vi "PumpValve4.vi"() -> ()   [LabVIEW 2015]
uses:
  PumpValve.ctl
  <vilib>/DAQmx/write.llb/DAQmx Write (Digital 1D Bool NChan 1Samp 1Line).vi
  <vilib>/DAQmx/miscellaneous.llb/DAQmx Fill In Error Info.vi
panel:
  in  "Duty cycle % (0-100)":dbl=50.0
  in  "stop":bool
  in  "Steps in a cycle":i32=256
  in  "Cycle time (s)":i32=5
  in  "On/Off (Pump)":bool
  in  "Open/Close (Blue)":bool
  in  "Open/Close (Green)":bool
  in  "Manual Mode":bool
  out "Invalid fill%":bool
  out "Tank":u32(slide) scale=0.0..100.0
  in  "Drain %":u32
  in  "Fill %":u32
  in  "Drain":bool
  in  "Stop Program":bool
  in  "Fill":bool
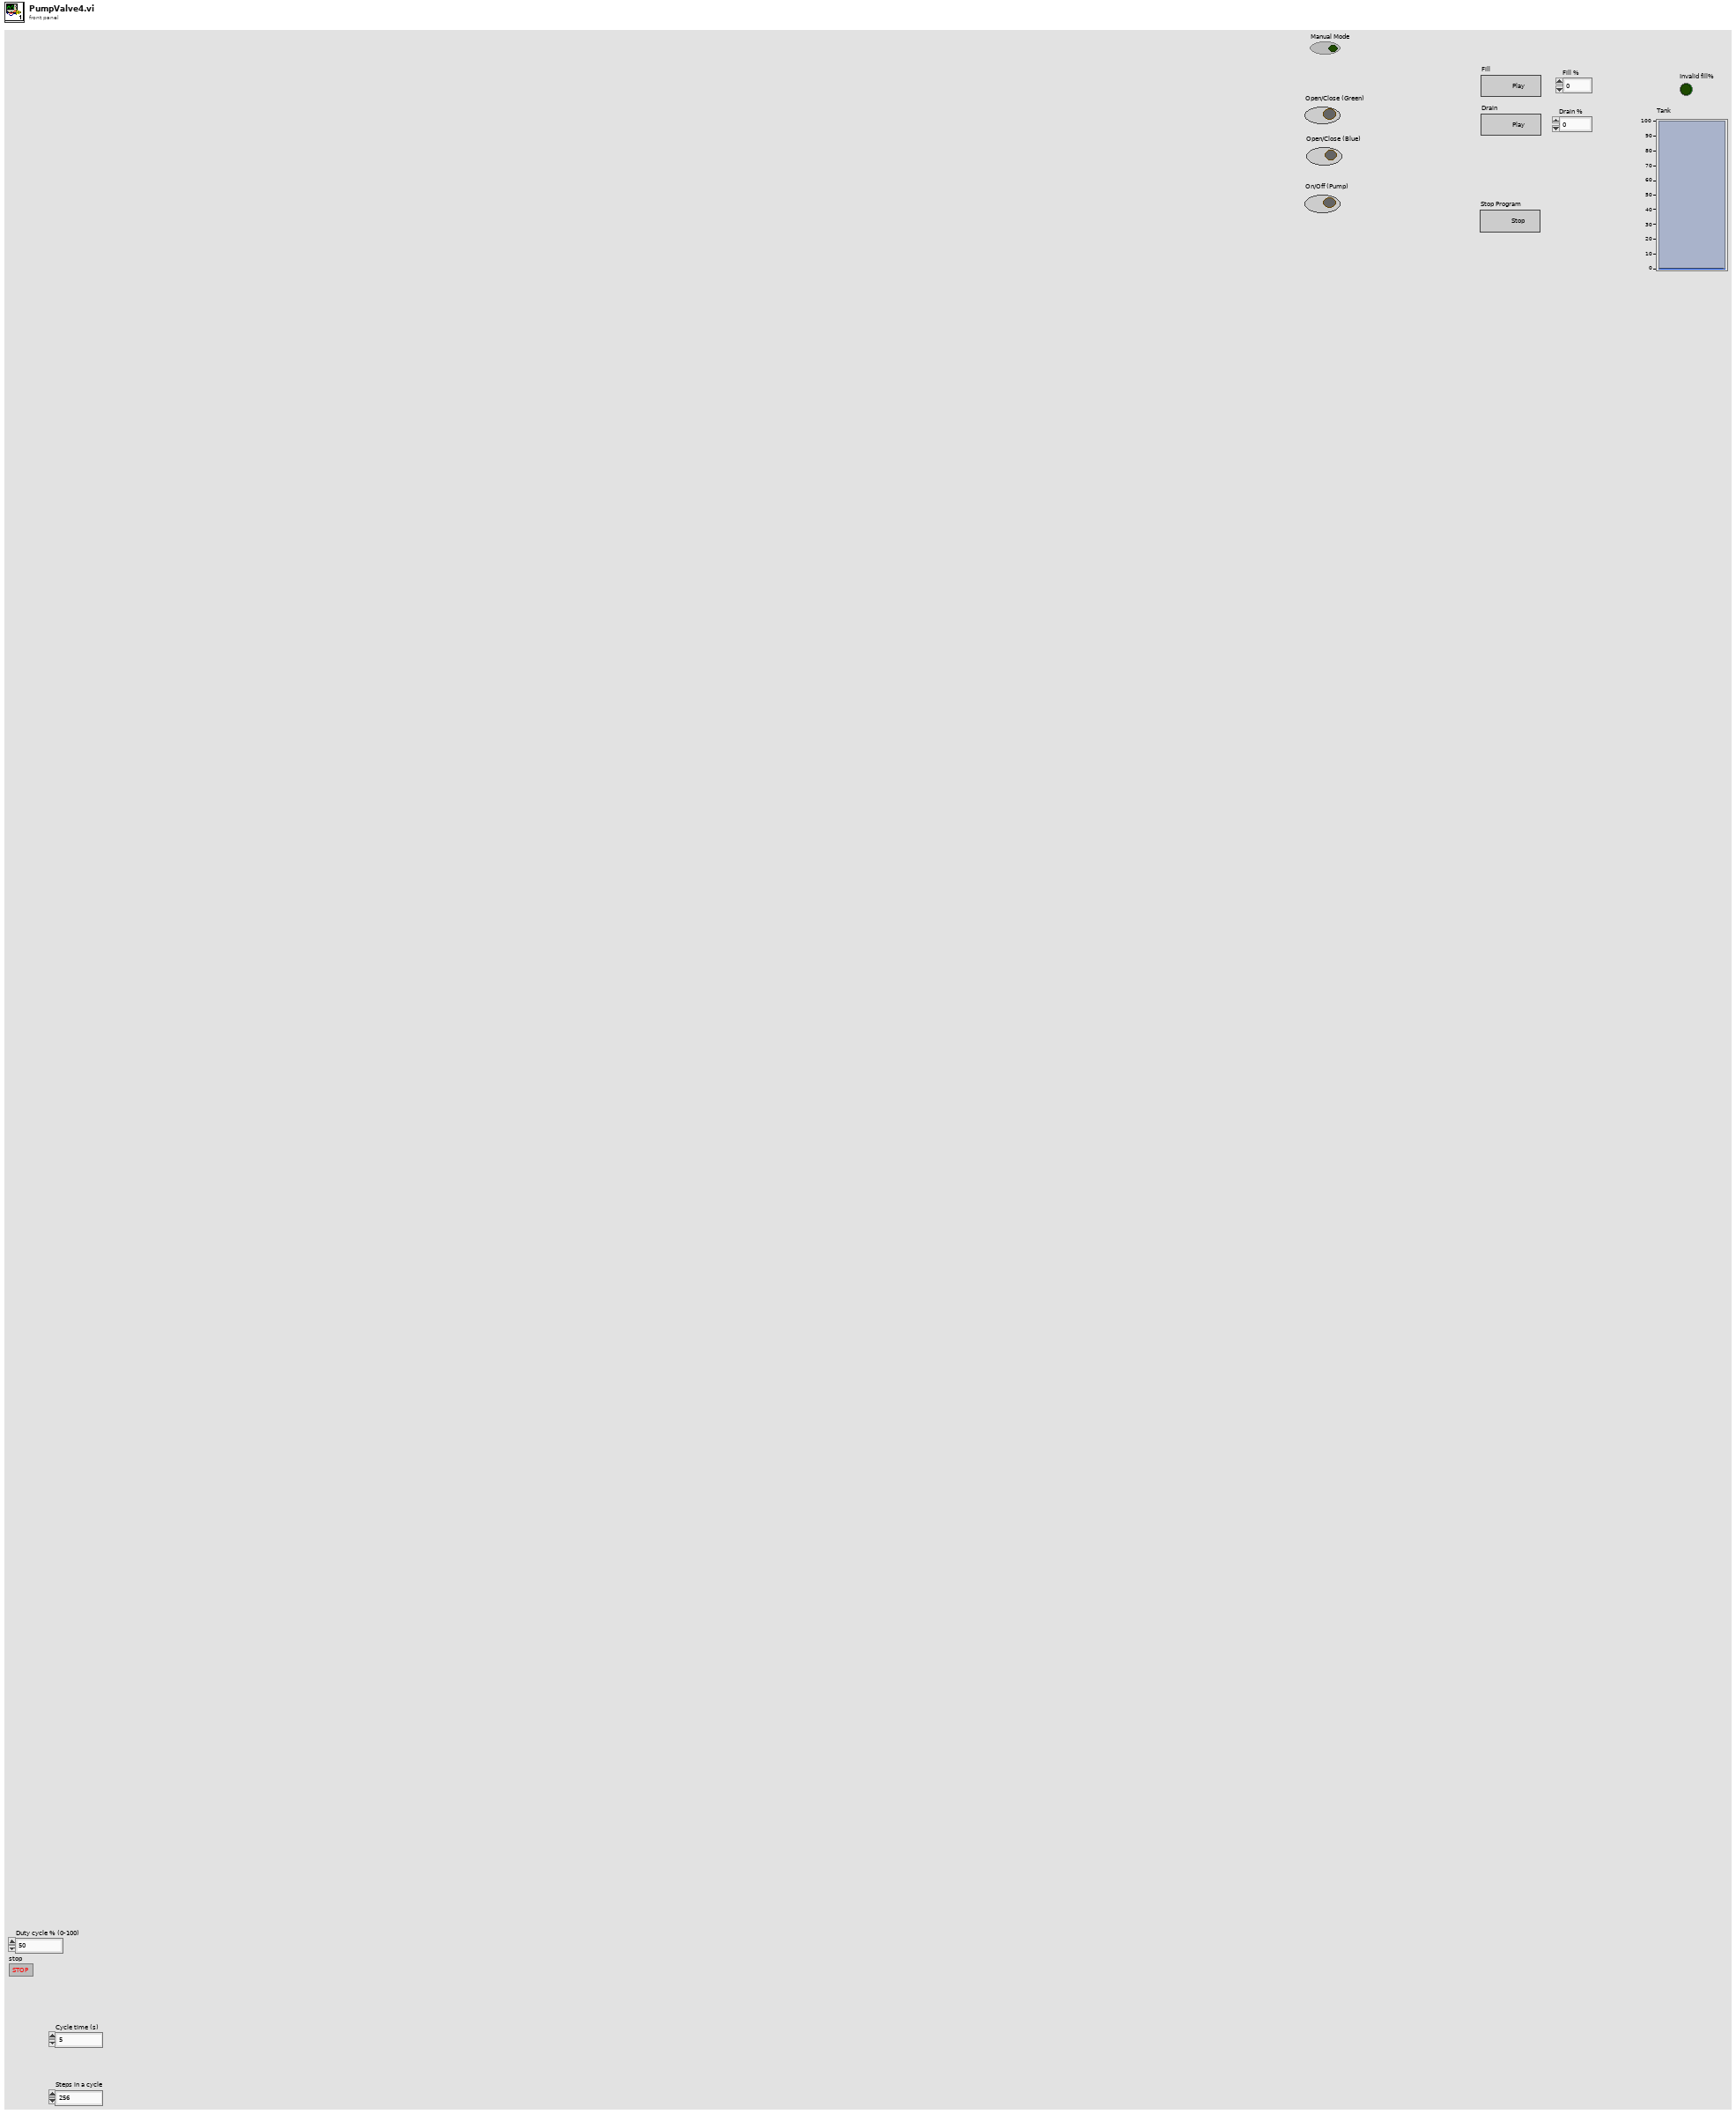
[diagram p1: front panel]
types:
  T1 = typedef "PumpValve.ctl" = enum16{"PressureSetting", "ManualPressure", "ManualTemp", "Idle Temp", "Set Temp", "Initialize", "Idle", "Fill", "Drain", "Stop"}
  T2 = cluster{"Open/Close (Green)":bool, "Open/Close (Blue)":bool, "On/Off (Pump)":bool}
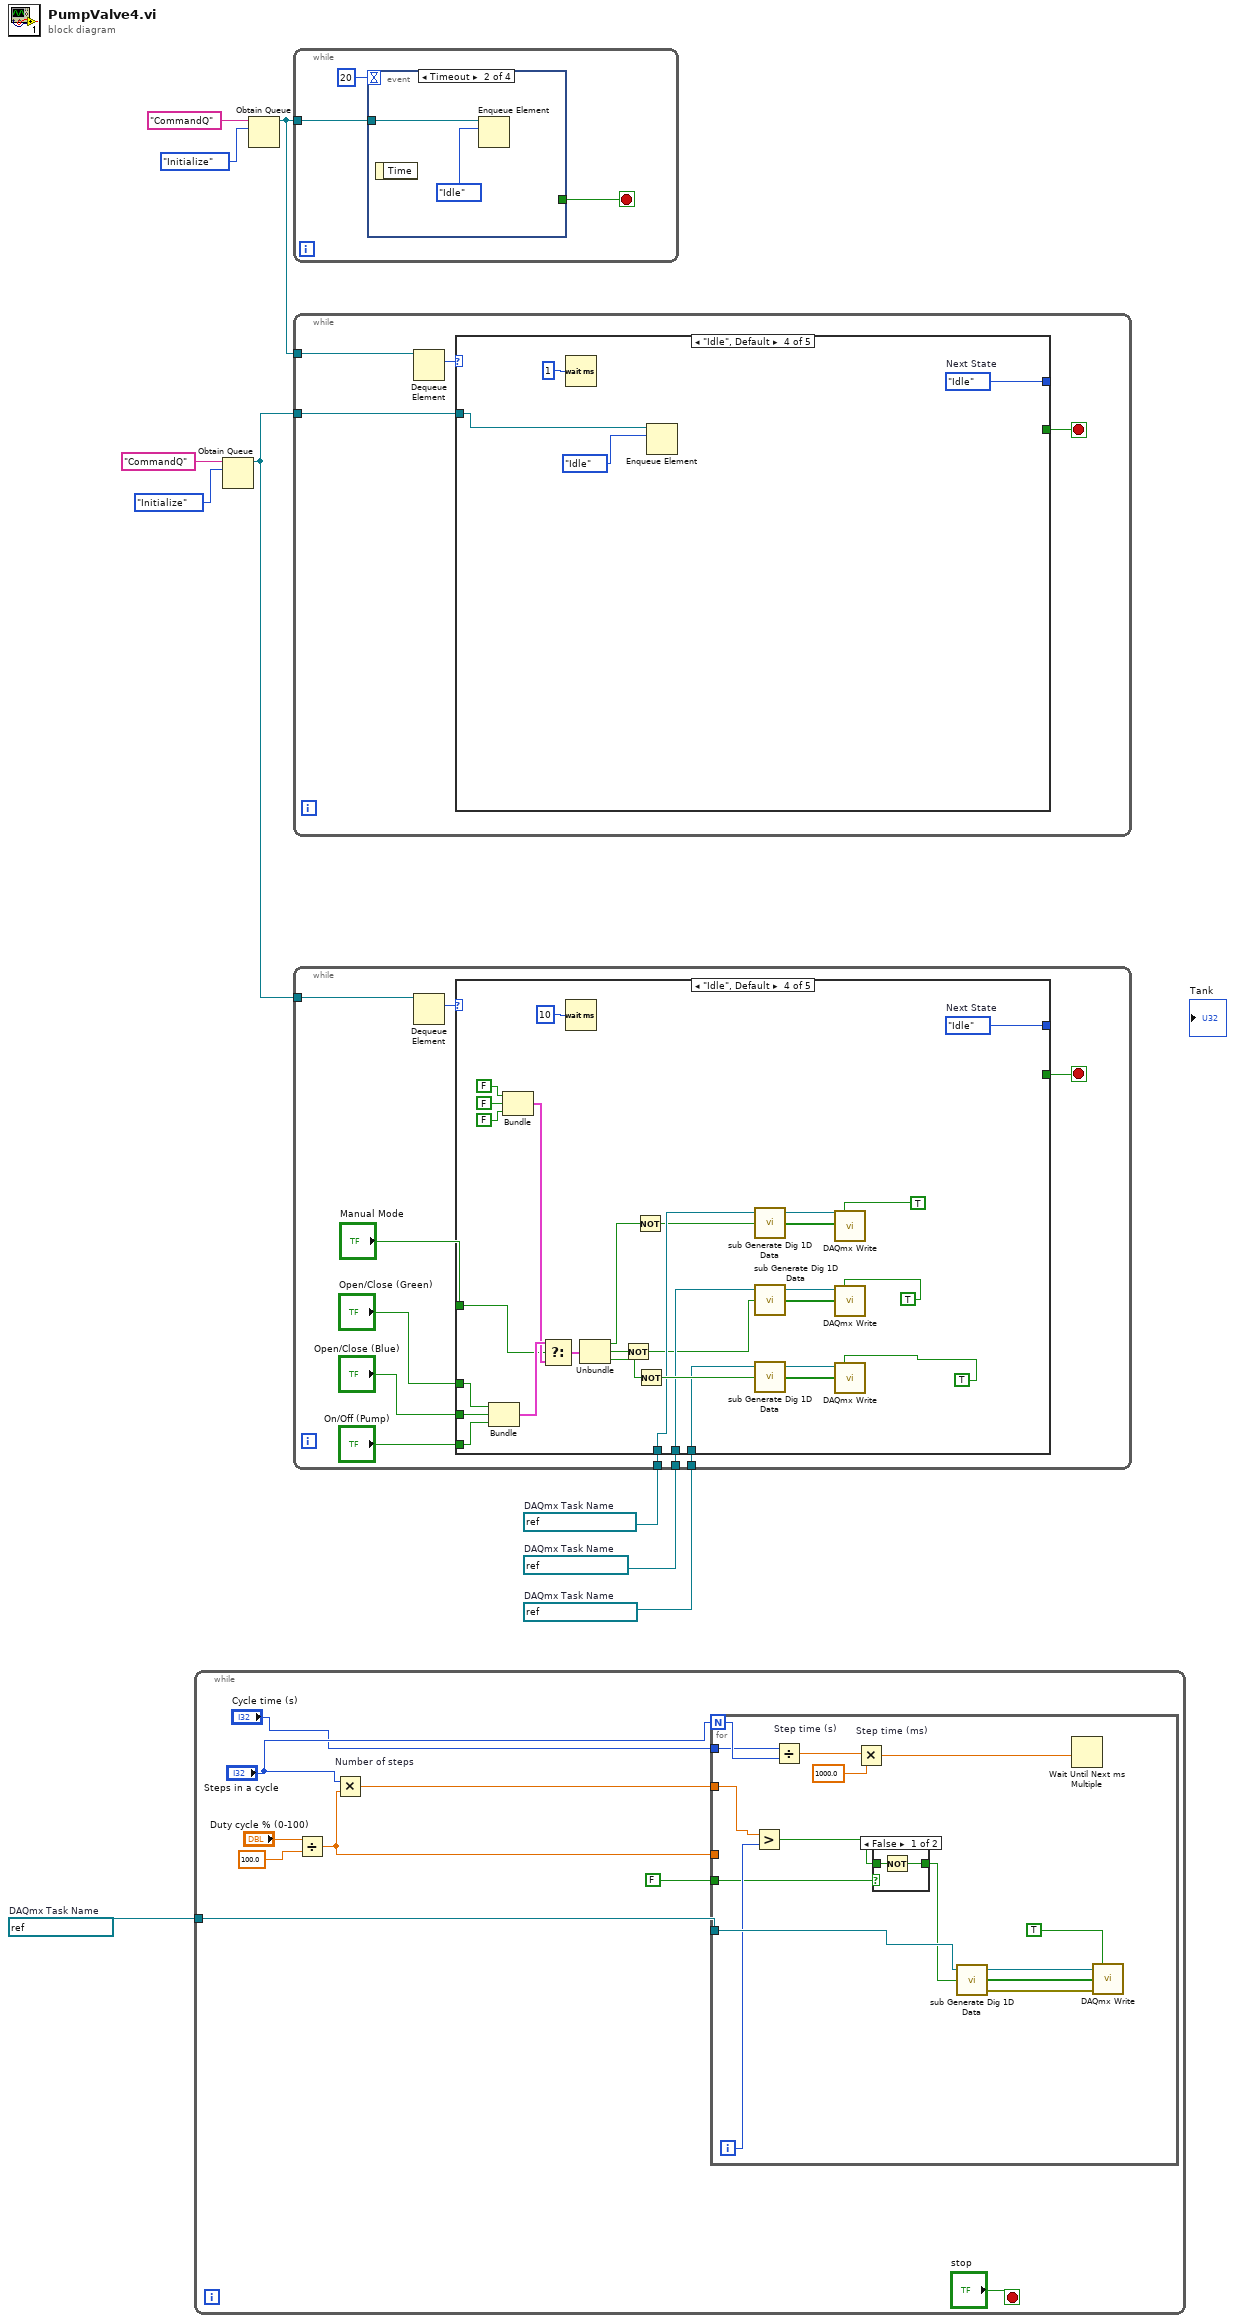
[diagram p0: block diagram]
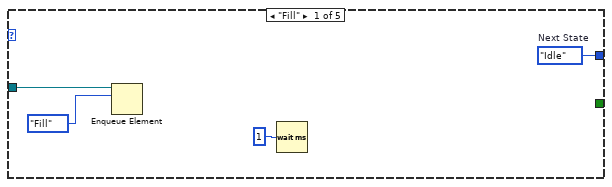
[diagram p3: hidden frame]
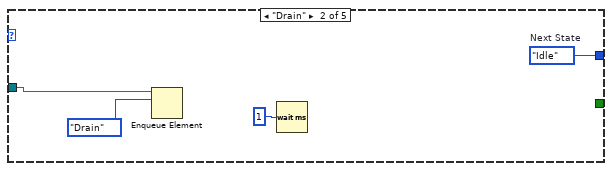
[diagram p4: hidden frame]
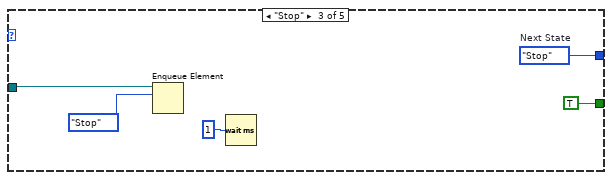
[diagram p5: hidden frame]
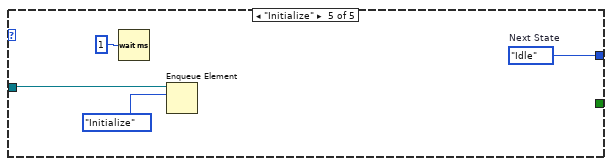
[diagram p6: hidden frame]
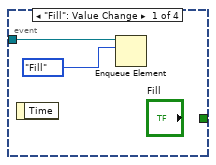
[diagram p7: hidden frame]
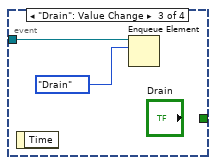
[diagram p8: hidden frame]
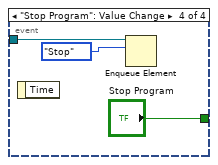
[diagram p9: hidden frame]
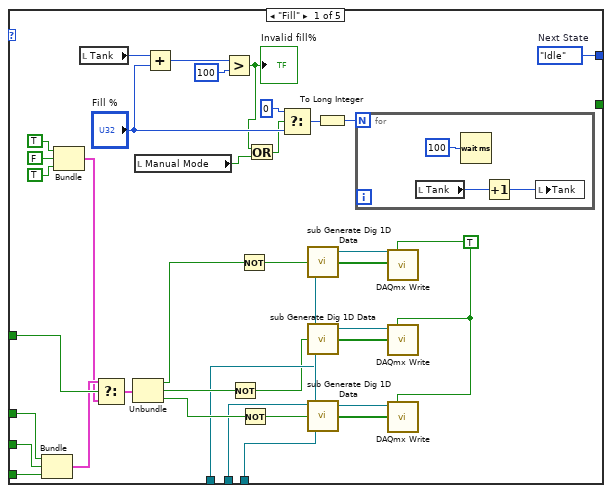
[diagram p10: hidden frame]
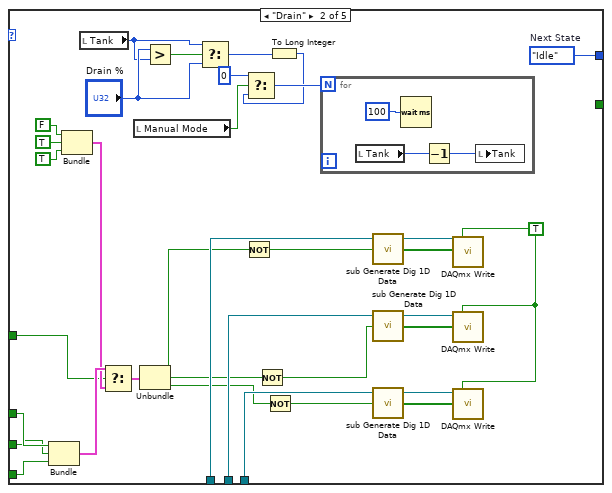
[diagram p11: hidden frame]
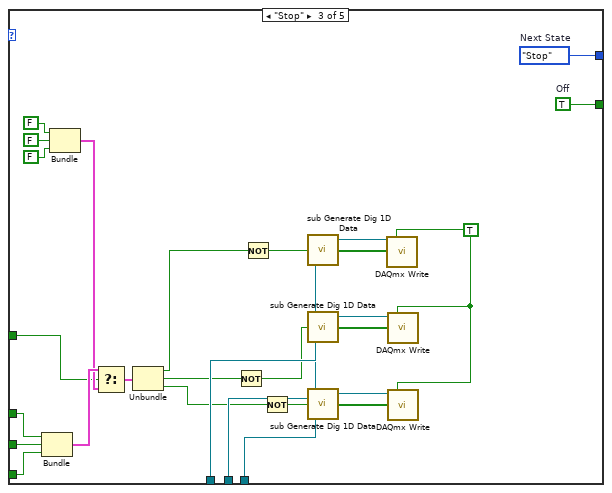
[diagram p12: hidden frame]
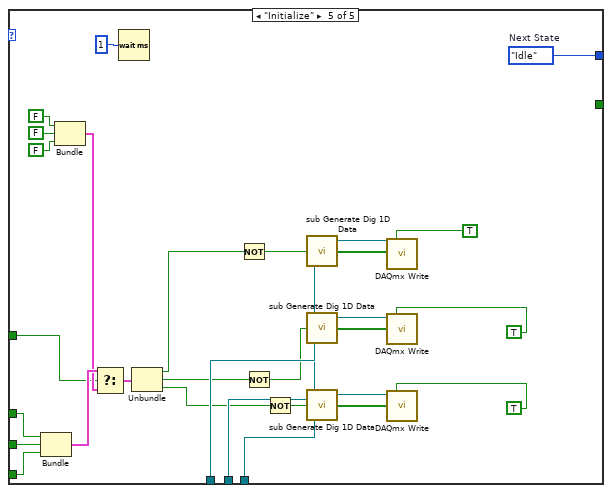
[diagram p13: hidden frame]
diagram:
  w1 = refnum<k21> "DigitalOutBlue"  # DAQmx Task Name
  w6 = refnum<k21> "PumpTask-P0L0"  # DAQmx Task Name
  w7 = refnum<k21> "BlueTask-P0L1"  # DAQmx Task Name
  w8 = refnum<k21> "GreenTask-P0L2"  # DAQmx Task Name
  n1 = while {
    tunnel: w1 -> [w19]
    stop <- "stop" stop-if-true
    n2 = Divide(x="Duty cycle % (0-100)", y=100.0) -> (x/y=w15:dbl)
    n3 = Multiply "Number of steps"(x="Steps in a cycle", y=w15) -> (x*y=w12:dbl)
    n4 = for {
      N: "Steps in a cycle" -> [w28]
      tunnel: w19 -> [w30]
      tunnel: w15 -> [_]
      tunnel: "Cycle time (s)" -> [w27]
      tunnel: w12 -> [w23]
      tunnel: FALSE -> [w20]
      i -> [w22]
      n5 = Greater?(x=w23, y=w22) -> (0:w21:bool)
      n6 = Divide "Step time (s)"(x=w27, y=w28) -> (x/y=w26:dbl)
      n7 = Multiply "Step time (ms)"(x=w26, y=1000.0) -> (x*y=w24:dbl)
      n8 = case shown="False" w20 {
        tunnel: [w35 w37] -> w29
        tunnel: w21 -> [w36 w37]
        frame False {
          n9 = Not(x=w36) -> (.not. x?=w35:bool)
        }
        frame True {
        }
      }
      n10 = call <vilib>:"sub Generate Dig 1D Data.vi"("initial value"=w29, "task in"=w30) -> ("error out"=w33:errorcluster, "Data"=w32:bool[], "task out"=w31:refnum<k21>)  [unwired: 1 in]
      n11 = Wait Until Next ms Multiple(millisecond multiple=w24) -> ()  [unwired: 1 out]
      n12 = call-poly <vilib>:"DAQmx Write.vi"("task/channels in"=w31, "auto start"=TRUE, "data"=w32, "error in"=w33) -> ()  [unwired: 9 in, 3 out]
    }
  }
  n13 = Obtain Queue(name (unnamed)="CommandQ", element data type=PumpValve."Initialize" ("States")) -> (queue out=w2:refnum<queue>)  [unwired: 3 in, 2 out]
  n14 = Obtain Queue(name (unnamed)="CommandQ", element data type=PumpValve."Initialize" ("States")) -> (queue out=w5:refnum<queue>)  [unwired: 3 in, 2 out]
  n15 = while {
    tunnel: w5 -> [w39]
    stop <- w38 stop-if-true
    n16 = event shown="[1] Timeout" {
      selector: _ -> [_ _ _ _]
      dyn-events: _ -> [_ _ _ _]
      timeout: 20 -> [_ _ _ _]
      tunnel: w39 -> [w42 w44 w46 w49]
      tunnel: [_ _ _ "Stop Program"] -> w38
      event "Fill": Value Change {
        n17 = event-data() -> ()  [unwired: 1 in, 1 out]
        n18 = Enqueue Element(queue=w42, element=PumpValve."Fill" ("States")) -> ()  [unwired: 2 in, 3 out]
      }
      event Timeout {
        n19 = event-data() -> ()  [unwired: 1 in, 1 out]
        n20 = Enqueue Element(queue=w44, element=PumpValve."Idle" ("States")) -> ()  [unwired: 2 in, 3 out]
      }
      event "Drain": Value Change {
        n21 = event-data() -> ()  [unwired: 1 in, 1 out]
        n22 = Enqueue Element(queue=w46, element=PumpValve."Drain" ("States")) -> ()  [unwired: 2 in, 3 out]
      }
      event "Stop Program": Value Change {
        n23 = event-data() -> ()  [unwired: 1 in, 1 out]
        n24 = Enqueue Element(queue=w49, element=PumpValve."Stop" ("States")) -> ()  [unwired: 2 in, 3 out]
      }
    }
  }
  n25 = while {
    tunnel: w5 -> [w52]
    tunnel: w2 -> [w51]
    stop <- w50 stop-if-true
    n26 = Dequeue Element(queue=w52) -> (element=w53:T1)  [unwired: 2 in, 3 out]
    n27 = case shown="\"Idle\", Default" w53 {
      tunnel: [w57 w61 w66 w70 w74] -> _
      tunnel: w51 -> [w54 w58 w63 w67 w71]
      tunnel: [_ _ TRUE _ _] -> w50
      frame "Fill" {
        w57 = PumpValve."Idle"  # Next State
        n28 = Enqueue Element(queue=w54, element=PumpValve."Fill" ("States")) -> ()  [unwired: 2 in, 3 out]
        n29 = Wait (ms)(milliseconds to wait=u32 1) -> ()  [unwired: 1 out]
      }
      frame "Drain" {
        w61 = PumpValve."Idle"  # Next State
        n30 = Enqueue Element(queue=w58, element=PumpValve."Drain" ("States")) -> ()  [unwired: 2 in, 3 out]
        n31 = Wait (ms)(milliseconds to wait=u32 1) -> ()  [unwired: 1 out]
      }
      frame "Stop" {
        w66 = PumpValve."Stop"  # Next State
        n32 = Enqueue Element(queue=w63, element=PumpValve."Stop" ("States")) -> ()  [unwired: 2 in, 3 out]
        n33 = Wait (ms)(milliseconds to wait=u32 1) -> ()  [unwired: 1 out]
      }
      frame "Idle", Default {
        w70 = PumpValve."Idle"  # Next State
        n34 = Wait (ms)(milliseconds to wait=u32 1) -> ()  [unwired: 1 out]
        n35 = Enqueue Element(queue=w67, element=PumpValve."Idle" ("States")) -> ()  [unwired: 2 in, 3 out]
      }
      frame "Initialize" {
        w74 = PumpValve."Idle"  # Next State
        n36 = Wait (ms)(milliseconds to wait=u32 1) -> ()  [unwired: 1 out]
        n37 = Enqueue Element(queue=w71, element=PumpValve."Initialize" ("States")) -> ()  [unwired: 2 in, 3 out]
      }
    }
  }
  n38 = while {
    tunnel: w2 -> [w84]
    tunnel: w8 -> [w75]
    tunnel: w7 -> [w76]
    tunnel: w6 -> [w77]
    stop <- w83 stop-if-true
    n39 = Dequeue Element(queue=w84) -> (element=w82:T1)  [unwired: 2 in, 3 out]
    n40 = case shown="\"Idle\", Default" w82 {
      tunnel: [w121 w159 w190 w220 w250] -> _
      tunnel: [_ _ w163 _ _] -> w83
      tunnel: "Open/Close (Blue)" -> [w107 w135 w171 w203 w230]
      tunnel: "Open/Close (Green)" -> [w106 w136 w172 w204 w231]
      tunnel: "On/Off (Pump)" -> [w105 w134 w170 w202 w229]
      tunnel: "Manual Mode" -> [w104 w137 w173 w205 w232]
      tunnel: w77 -> [w90 w131 w175 w195 w234]
      tunnel: w76 -> [w89 w132 w176 w194 w235]
      tunnel: w75 -> [w88 w133 w177 w193 w236]
      frame "Fill" {
        w100 = TRUE
        w121 = PumpValve."Idle"  # Next State
        n41 = Bundle("Open/Close (Green)"=w106, "Open/Close (Blue)"=w107, "On/Off (Pump)"=w105) -> (w103:T2)  [unwired: 1 in]
        n42 = Bundle(TRUE, FALSE, TRUE) -> (w102:cluster{bool, bool, bool})  [unwired: 1 in]
        n43 = local read "Tank"() -> (w120:u32)
        n44 = Select(t=w103, s=w104, f=w102) -> (s? t:f=w101:T2)
        n45 = Unbundle(w101) -> ("Open/Close (Green)"=w93:bool, "Open/Close (Blue)"=w92:bool, "On/Off (Pump)"=w91:bool)
        n46 = local read "Manual Mode"() -> (w109:bool)
        n47 = Add(x=w120, y="Fill %") -> (x+y=w118:u32)
        n48 = Greater?(x=w118, y=u32 100) -> (0:w110:bool)
        "Invalid fill%" <- w110
        n49 = Not(x=w92) -> (.not. x?=w85:bool)
        n50 = Not(x=w93) -> (.not. x?=w86:bool)
        n51 = Not(x=w91) -> (.not. x?=w87:bool)
        n52 = Or(x=w110, y=w109) -> (x .or. y?=w108:bool)
        n53 = Select(t=u32 0, s=w108, f="Fill %") -> (s? t:f=w115:u32)
        n54 = call <vilib>:"sub Generate Dig 1D Data.vi"("initial value"=w86, "task in"=w88) -> ("Data"=w95:bool[], "task out"=w99:refnum<k21>)  [unwired: 1 in, 1 out]
        n55 = call <vilib>:"sub Generate Dig 1D Data.vi"("initial value"=w85, "task in"=w89) -> ("Data"=w96:bool[], "task out"=w98:refnum<k21>)  [unwired: 1 in, 1 out]
        n56 = call <vilib>:"sub Generate Dig 1D Data.vi"("initial value"=w87, "task in"=w90) -> ("Data"=w94:bool[], "task out"=w97:refnum<k21>)  [unwired: 1 in, 1 out]
        n57 = To Long Integer(number=w115) -> (32bit integer=w114:i32)
        n58 = for {
          N: w114 -> [_]
          n59 = local read "Tank"() -> (w124:u32)
          n60 = Wait (ms)(milliseconds to wait=u32 100 ("y")) -> ()  [unwired: 1 out]
          n61 = Increment(x=w124) -> (x+1=w123:u32)
          n62 = local write "Tank"(w123) -> ()
        }
        n63 = call-poly <vilib>:"DAQmx Write.vi"("task/channels in"=w99, "auto start"=w100, "data"=w95) -> ()  [unwired: 10 in, 3 out]
        n64 = call-poly <vilib>:"DAQmx Write.vi"("task/channels in"=w98, "auto start"=w100, "data"=w96) -> ()  [unwired: 10 in, 3 out]
        n65 = call-poly <vilib>:"DAQmx Write.vi"("task/channels in"=w97, "auto start"=w100, "data"=w94) -> ()  [unwired: 10 in, 3 out]
      }
      frame "Drain" {
        w141 = TRUE
        w159 = PumpValve."Idle"  # Next State
        n66 = Bundle("Open/Close (Green)"=w136, "Open/Close (Blue)"=w135, "On/Off (Pump)"=w134) -> (w139:T2)  [unwired: 1 in]
        n67 = Bundle(FALSE, TRUE, TRUE) -> (w138:cluster{bool, bool, bool})  [unwired: 1 in]
        n68 = local read "Tank"() -> (w156:u32)
        n69 = Select(t=w139, s=w137, f=w138) -> (s? t:f=w140:T2)
        n70 = local read "Manual Mode"() -> (w151:bool)
        n71 = Unbundle(w140) -> ("Open/Close (Green)"=w130:bool, "Open/Close (Blue)"=w129:bool, "On/Off (Pump)"=w128:bool)
        n72 = Greater?(x="Drain %", y=w156) -> (0:w152:bool)
        n73 = Select(t=w156, s=w152, f="Drain %") -> (s? t:f=w158:u32)
        n74 = Not(x=w130) -> (.not. x?=w126:bool)
        n75 = Not(x=w129) -> (.not. x?=w125:bool)
        n76 = Not(x=w128) -> (.not. x?=w127:bool)
        n77 = To Long Integer(number=w158) -> (32bit integer=w148:i32)
        n78 = Select(t=0, s=w151, f=w148) -> (s? t:f=w149:i32)
        n79 = for {
          N: w149 -> [_]
          n80 = local read "Tank"() -> (w161:u32)
          n81 = Wait (ms)(milliseconds to wait=u32 100) -> ()  [unwired: 1 out]
          n82 = Decrement(x=w161) -> (x-1=w162:u32)
          n83 = local write "Tank"(w162) -> ()
        }
        n84 = call <vilib>:"sub Generate Dig 1D Data.vi"("initial value"=w126, "task in"=w133) -> ("Data"=w146:bool[], "task out"=w142:refnum<k21>)  [unwired: 1 in, 1 out]
        n85 = call <vilib>:"sub Generate Dig 1D Data.vi"("initial value"=w125, "task in"=w132) -> ("Data"=w145:bool[], "task out"=w143:refnum<k21>)  [unwired: 1 in, 1 out]
        n86 = call <vilib>:"sub Generate Dig 1D Data.vi"("initial value"=w127, "task in"=w131) -> ("Data"=w147:bool[], "task out"=w144:refnum<k21>)  [unwired: 1 in, 1 out]
        n87 = call-poly <vilib>:"DAQmx Write.vi"("task/channels in"=w142, "auto start"=w141, "data"=w146) -> ()  [unwired: 10 in, 3 out]
        n88 = call-poly <vilib>:"DAQmx Write.vi"("task/channels in"=w143, "auto start"=w141, "data"=w145) -> ()  [unwired: 10 in, 3 out]
        n89 = call-poly <vilib>:"DAQmx Write.vi"("task/channels in"=w144, "auto start"=w141, "data"=w147) -> ()  [unwired: 10 in, 3 out]
      }
      frame "Stop" {
        w184 = TRUE
        w163 = TRUE  # Off
        w190 = PumpValve."Stop"  # Next State
        n90 = Bundle("Open/Close (Green)"=w172, "Open/Close (Blue)"=w171, "On/Off (Pump)"=w170) -> (w186:T2)  [unwired: 1 in]
        n91 = Bundle(FALSE, FALSE, FALSE) -> (w174:cluster{bool, bool, bool})  [unwired: 1 in]
        n92 = Select(t=w186, s=w173, f=w174) -> (s? t:f=w185:T2)
        n93 = Unbundle(w185) -> ("Open/Close (Green)"=w169:bool, "Open/Close (Blue)"=w168:bool, "On/Off (Pump)"=w167:bool)
        n94 = Not(x=w168) -> (.not. x?=w164:bool)
        n95 = Not(x=w169) -> (.not. x?=w165:bool)
        n96 = Not(x=w167) -> (.not. x?=w166:bool)
        n97 = call <vilib>:"sub Generate Dig 1D Data.vi"("initial value"=w165, "task in"=w177) -> ("Data"=w179:bool[], "task out"=w183:refnum<k21>)  [unwired: 1 in, 1 out]
        n98 = call <vilib>:"sub Generate Dig 1D Data.vi"("initial value"=w164, "task in"=w176) -> ("Data"=w180:bool[], "task out"=w182:refnum<k21>)  [unwired: 1 in, 1 out]
        n99 = call <vilib>:"sub Generate Dig 1D Data.vi"("initial value"=w166, "task in"=w175) -> ("Data"=w178:bool[], "task out"=w181:refnum<k21>)  [unwired: 1 in, 1 out]
        n100 = call-poly <vilib>:"DAQmx Write.vi"("task/channels in"=w183, "auto start"=w184, "data"=w179) -> ()  [unwired: 10 in, 3 out]
        n101 = call-poly <vilib>:"DAQmx Write.vi"("task/channels in"=w182, "auto start"=w184, "data"=w180) -> ()  [unwired: 10 in, 3 out]
        n102 = call-poly <vilib>:"DAQmx Write.vi"("task/channels in"=w181, "auto start"=w184, "data"=w178) -> ()  [unwired: 10 in, 3 out]
      }
      frame "Idle", Default {
        w220 = PumpValve."Idle"  # Next State
        n103 = Bundle("Open/Close (Green)"=w204, "Open/Close (Blue)"=w203, "On/Off (Pump)"=w202) -> (w215:T2)  [unwired: 1 in]
        n104 = Bundle(FALSE, FALSE, FALSE) -> (w206:cluster{bool, bool, bool})  [unwired: 1 in]
        n105 = Select(t=w215, s=w205, f=w206) -> (s? t:f=w214:T2)
        n106 = Wait (ms)(milliseconds to wait=u32 10) -> ()  [unwired: 1 out]
        n107 = Unbundle(w214) -> ("Open/Close (Green)"=w201:bool, "Open/Close (Blue)"=w200:bool, "On/Off (Pump)"=w199:bool)
        n108 = Not(x=w200) -> (.not. x?=w191:bool)
        n109 = Not(x=w201) -> (.not. x?=w192:bool)
        n110 = Not(x=w199) -> (.not. x?=w198:bool)
        n111 = call <vilib>:"sub Generate Dig 1D Data.vi"("initial value"=w192, "task in"=w193) -> ("Data"=w208:bool[], "task out"=w212:refnum<k21>)  [unwired: 1 in, 1 out]
        n112 = call <vilib>:"sub Generate Dig 1D Data.vi"("initial value"=w191, "task in"=w194) -> ("Data"=w209:bool[], "task out"=w211:refnum<k21>)  [unwired: 1 in, 1 out]
        n113 = call <vilib>:"sub Generate Dig 1D Data.vi"("initial value"=w198, "task in"=w195) -> ("Data"=w207:bool[], "task out"=w210:refnum<k21>)  [unwired: 1 in, 1 out]
        n114 = call-poly <vilib>:"DAQmx Write.vi"("task/channels in"=w212, "auto start"=TRUE, "data"=w208) -> ()  [unwired: 10 in, 3 out]
        n115 = call-poly <vilib>:"DAQmx Write.vi"("task/channels in"=w211, "auto start"=TRUE, "data"=w209) -> ()  [unwired: 10 in, 3 out]
        n116 = call-poly <vilib>:"DAQmx Write.vi"("task/channels in"=w210, "auto start"=TRUE, "data"=w207) -> ()  [unwired: 10 in, 3 out]
      }
      frame "Initialize" {
        w250 = PumpValve."Idle"  # Next State
        n117 = Bundle("Open/Close (Green)"=w231, "Open/Close (Blue)"=w230, "On/Off (Pump)"=w229) -> (w245:T2)  [unwired: 1 in]
        n118 = Bundle(FALSE, FALSE, FALSE) -> (w233:cluster{bool, bool, bool})  [unwired: 1 in]
        n119 = Select(t=w245, s=w232, f=w233) -> (s? t:f=w244:T2)
        n120 = Wait (ms)(milliseconds to wait=u32 1) -> ()  [unwired: 1 out]
        n121 = Unbundle(w244) -> ("Open/Close (Green)"=w228:bool, "Open/Close (Blue)"=w227:bool, "On/Off (Pump)"=w226:bool)
        n122 = Not(x=w228) -> (.not. x?=w222:bool)
        n123 = Not(x=w227) -> (.not. x?=w221:bool)
        n124 = Not(x=w226) -> (.not. x?=w225:bool)
        n125 = call <vilib>:"sub Generate Dig 1D Data.vi"("initial value"=w222, "task in"=w236) -> ("Data"=w238:bool[], "task out"=w242:refnum<k21>)  [unwired: 1 in, 1 out]
        n126 = call <vilib>:"sub Generate Dig 1D Data.vi"("initial value"=w221, "task in"=w235) -> ("Data"=w239:bool[], "task out"=w241:refnum<k21>)  [unwired: 1 in, 1 out]
        n127 = call <vilib>:"sub Generate Dig 1D Data.vi"("initial value"=w225, "task in"=w234) -> ("Data"=w237:bool[], "task out"=w240:refnum<k21>)  [unwired: 1 in, 1 out]
        n128 = call-poly <vilib>:"DAQmx Write.vi"("task/channels in"=w242, "auto start"=TRUE, "data"=w238) -> ()  [unwired: 10 in, 3 out]
        n129 = call-poly <vilib>:"DAQmx Write.vi"("task/channels in"=w241, "auto start"=TRUE, "data"=w239) -> ()  [unwired: 10 in, 3 out]
        n130 = call-poly <vilib>:"DAQmx Write.vi"("task/channels in"=w240, "auto start"=TRUE, "data"=w237) -> ()  [unwired: 10 in, 3 out]
      }
    }
  }
